vi "Create New File.vi"(8 "error in (no error)":errorcluster, 10 "Path":path, 11 "File Manager in":refnum<class "File Abstract.lvclass">) -> (0 "error out":errorcluster, 1 "Path out":path, 2 "File Refnum":variant, 3 "File Manager out":refnum<class "File Abstract.lvclass">)   [LabVIEW 2021, in "File Abstract.lvclass"]
doc: "This VI helps to save file path into class data (File Abstract.ctl)"
uses:
  File Abstract.lvclass
  File Abstract.lvclass/File Abstract.ctl
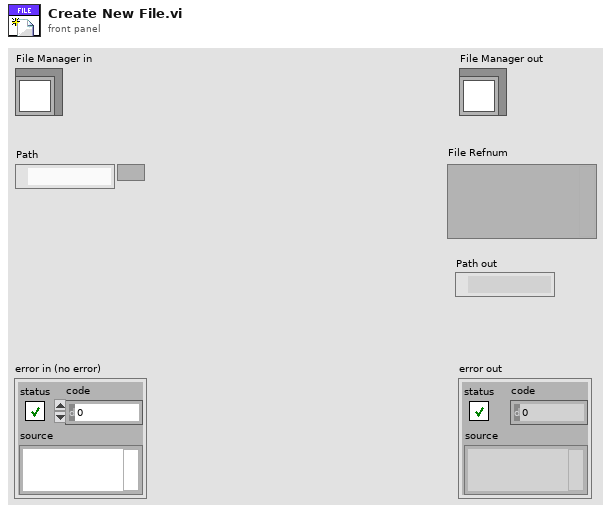
[diagram p1: front panel]
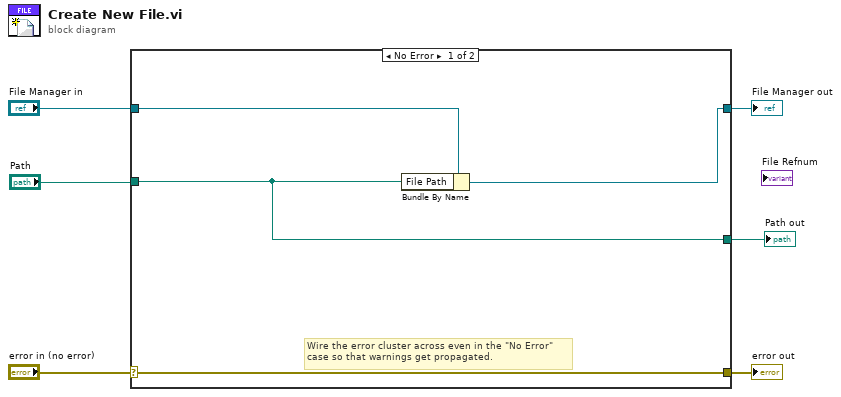
[diagram p0: block diagram]
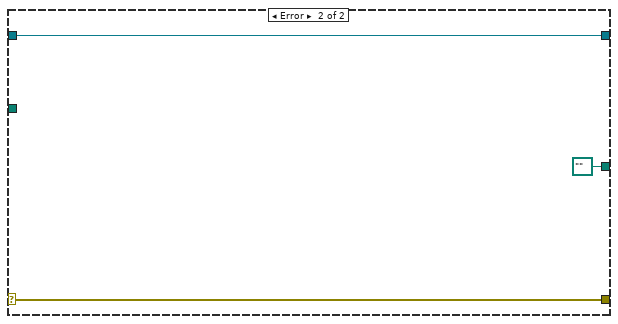
[diagram p2: hidden frame]
diagram:
  n1 = case shown="No Error" "error in (no error)" {
    selector: "error in (no error)" -> [w10 w13]
    tunnel: [w10 w13] -> w5
    tunnel: [w8 w12] -> w3
    tunnel: "File Manager in" -> [w9 w12]
    tunnel: "Path" -> [w7 _]
    tunnel: [w7 path "" ("Path")] -> w1
    frame No Error {
      # "Wire the error cluster across even in the \"No Error\"\ncase so that warnings get propagated."
      n2 = Bundle By Name(cluster=w9, "File Path"=w7) -> (w8:refnum<class "File Abstract.lvclass">)
    }
    frame Error {
    }
  }
  "error out" <- w5
  "File Manager out" <- w3
  "Path out" <- w1
